vi "DO Write.vi"(8 "error in (no error)":errorcluster, 10 "Digital Output":bool, 11 "TCP 380 in":refnum<class "TCP 380.lvclass">) -> (0 "error out":errorcluster)   [LabVIEW 2021, in "TCP 380.lvclass"]
uses:
  TCP 380.lvclass
  TCP 380.lvclass/TCP 380.ctl
  <vilib>/NathanCo/Digital-Tasks/Digital Output/Digital Output/Digital Output.lvclass
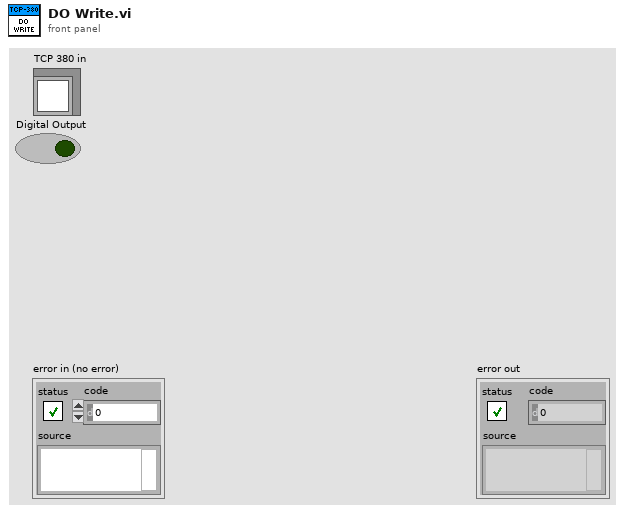
[diagram p1: front panel]
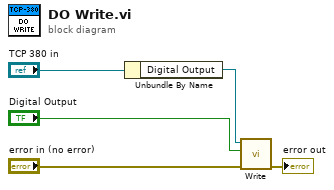
[diagram p0: block diagram]
diagram:
  n1 = Unbundle By Name("TCP 380 in") -> ("Digital Output"=w1:refnum<class "Digital Output.lvclass">)
  n2 = call <vilib>:"Write.vi"("error in (no error)"="error in (no error)", "Digital Output"="Digital Output", "Digital Output in"=w1) -> ("error out"=→"error out":errorcluster)  [unwired: 8 in]
